vi "Facade.vi"(0 "Data In":T10 {"Input sources" items=["--unused--", "Probe Mic Right", "Probe Mic Left", "Cal Mic", "ABR", "CAP Right", "CAP Left", "Startle piezo", "Temperature", "Heart rate", "Accelerometer", "Startle piezo 2"]; "Output sources" items=["--unused--", "Right primary", "Right secondary", "Left primary", "Left secondary", "Shocks", "Startle", "Background", "Shaker", "Blue laser"]}, 2 "Display State In":T7, 3 "Container State":T9) -> (6 "Data Out":T10 {"Input sources" items=["--unused--", "Probe Mic Right", "Probe Mic Left", "Cal Mic", "ABR", "CAP Right", "CAP Left", "Startle piezo", "Temperature", "Heart rate", "Accelerometer", "Startle piezo 2"]; "Output sources" items=["--unused--", "Right primary", "Right secondary", "Left primary", "Left secondary", "Shocks", "Startle", "Background", "Shaker", "Blue laser"]}, 7 "Display State Out":T7, 8 "Action":T6)   [LabVIEW 2020, in "PXISlot.xctl"]
uses:
  PXISlot.xctl
  Input sources.ctl
  Output sources.ctl
  Data.ctl
  <vilib>/_xctls/Container State.ctl
  State.ctl
  Connector Type.ctl
  <vilib>/_xctls/Action.ctl
  <vilib>/_xctls/XControlSupport.lvlib
panel:
  in  "PXISlot Control":T1(tab) caption="SLOT X"
  in  "PXI-4461":cluster{"AI0":T2, "AO0":T3, "AO1":T3, "AI1":T2} caption="Slot X" {"AI1" items=["--unused--", "Probe Mic Right", "Probe Mic Left", "Cal Mic", "ABR", "CAP Right", "CAP Left", "Startle piezo", "Temperature", "Heart rate", "Accelerometer", "Startle piezo 2"]; "AO1" items=["--unused--", "Right primary", "Right secondary", "Left primary", "Left secondary", "Shocks", "Startle", "Background", "Shaker", "Blue laser"]; "AO0" items=["--unused--", "Right primary", "Right secondary", "Left primary", "Left secondary", "Shocks", "Startle", "Background", "Shaker", "Blue laser"]; "AI0" items=["--unused--", "Probe Mic Right", "Probe Mic Left", "Cal Mic", "ABR", "CAP Right", "CAP Left", "Startle piezo", "Temperature", "Heart rate", "Accelerometer", "Startle piezo 2"]}
  in  "BNC-2110":T4 caption="Slot X" {"AI7" items=["--unused--", "Probe Mic Right", "Probe Mic Left", "Cal Mic", "ABR", "CAP Right", "CAP Left", "Startle piezo", "Temperature", "Heart rate", "Accelerometer", "Startle piezo 2"]; "AI6" items=["--unused--", "Probe Mic Right", "Probe Mic Left", "Cal Mic", "ABR", "CAP Right", "CAP Left", "Startle piezo", "Temperature", "Heart rate", "Accelerometer", "Startle piezo 2"]; "AI5" items=["--unused--", "Probe Mic Right", "Probe Mic Left", "Cal Mic", "ABR", "CAP Right", "CAP Left", "Startle piezo", "Temperature", "Heart rate", "Accelerometer", "Startle piezo 2"]; "AI4" items=["--unused--", "Probe Mic Right", "Probe Mic Left", "Cal Mic", "ABR", "CAP Right", "CAP Left", "Startle piezo", "Temperature", "Heart rate", "Accelerometer", "Startle piezo 2"]; "AI3" items=["--unused--", "Probe Mic Right", "Probe Mic Left", "Cal Mic", "ABR", "CAP Right", "CAP Left", "Startle piezo", "Temperature", "Heart rate", "Accelerometer", "Startle piezo 2"]; "AI2" items=["--unused--", "Probe Mic Right", "Probe Mic Left", "Cal Mic", "ABR", "CAP Right", "CAP Left", "Startle piezo", "Temperature", "Heart rate", "Accelerometer", "Startle piezo 2"]; "AI1" items=["--unused--", "Probe Mic Right", "Probe Mic Left", "Cal Mic", "ABR", "CAP Right", "CAP Left", "Startle piezo", "Temperature", "Heart rate", "Accelerometer", "Startle piezo 2"]; "AO0" items=["--unused--", "Right primary", "Right secondary", "Left primary", "Left secondary", "Shocks", "Startle", "Background", "Shaker", "Blue laser"]; "AO1" items=["--unused--", "Right primary", "Right secondary", "Left primary", "Left secondary", "Shocks", "Startle", "Background", "Shaker", "Blue laser"]; "AI0" items=["--unused--", "Probe Mic Right", "Probe Mic Left", "Cal Mic", "ABR", "CAP Right", "CAP Left", "Startle piezo", "Temperature", "Heart rate", "Accelerometer", "Startle piezo 2"]}
  in  "BNC-2090":T5 caption="Slot X" {"AI7" items=["--unused--", "Probe Mic Right", "Probe Mic Left", "Cal Mic", "ABR", "CAP Right", "CAP Left", "Startle piezo", "Temperature", "Heart rate", "Accelerometer", "Startle piezo 2"]; "AI5" items=["--unused--", "Probe Mic Right", "Probe Mic Left", "Cal Mic", "ABR", "CAP Right", "CAP Left", "Startle piezo", "Temperature", "Heart rate", "Accelerometer", "Startle piezo 2"]; "AI3" items=["--unused--", "Probe Mic Right", "Probe Mic Left", "Cal Mic", "ABR", "CAP Right", "CAP Left", "Startle piezo", "Temperature", "Heart rate", "Accelerometer", "Startle piezo 2"]; "AI1" items=["--unused--", "Probe Mic Right", "Probe Mic Left", "Cal Mic", "ABR", "CAP Right", "CAP Left", "Startle piezo", "Temperature", "Heart rate", "Accelerometer", "Startle piezo 2"]; "AI6" items=["--unused--", "Probe Mic Right", "Probe Mic Left", "Cal Mic", "ABR", "CAP Right", "CAP Left", "Startle piezo", "Temperature", "Heart rate", "Accelerometer", "Startle piezo 2"]; "AI4" items=["--unused--", "Probe Mic Right", "Probe Mic Left", "Cal Mic", "ABR", "CAP Right", "CAP Left", "Startle piezo", "Temperature", "Heart rate", "Accelerometer", "Startle piezo 2"]; "AO1" items=["--unused--", "Right primary", "Right secondary", "Left primary", "Left secondary", "Shocks", "Startle", "Background", "Shaker", "Blue laser"]; "AI2" items=["--unused--", "Probe Mic Right", "Probe Mic Left", "Cal Mic", "ABR", "CAP Right", "CAP Left", "Startle piezo", "Temperature", "Heart rate", "Accelerometer", "Startle piezo 2"]; "AO0" items=["--unused--", "Right primary", "Right secondary", "Left primary", "Left secondary", "Shocks", "Startle", "Background", "Shaker", "Blue laser"]; "AI0" items=["--unused--", "Probe Mic Right", "Probe Mic Left", "Cal Mic", "ABR", "CAP Right", "CAP Left", "Startle piezo", "Temperature", "Heart rate", "Accelerometer", "Startle piezo 2"]}
  in  "PXIe-4463":cluster{"AO0":T3, "AO1":T3} caption="Slot X" {"AO1" items=["--unused--", "Right primary", "Right secondary", "Left primary", "Left secondary", "Shocks", "Startle", "Background", "Shaker", "Blue laser"]; "AO0" items=["--unused--", "Right primary", "Right secondary", "Left primary", "Left secondary", "Shocks", "Startle", "Background", "Shaker", "Blue laser"]}
  in  "PXIe-4464":cluster{"AI0":T2, "AI1":T2, "AI2":T2, "AI3":T2} caption="Slot X" {"AI3" items=["--unused--", "Probe Mic Right", "Probe Mic Left", "Cal Mic", "ABR", "CAP Right", "CAP Left", "Startle piezo", "Temperature", "Heart rate", "Accelerometer", "Startle piezo 2"]; "AI2" items=["--unused--", "Probe Mic Right", "Probe Mic Left", "Cal Mic", "ABR", "CAP Right", "CAP Left", "Startle piezo", "Temperature", "Heart rate", "Accelerometer", "Startle piezo 2"]; "AI1" items=["--unused--", "Probe Mic Right", "Probe Mic Left", "Cal Mic", "ABR", "CAP Right", "CAP Left", "Startle piezo", "Temperature", "Heart rate", "Accelerometer", "Startle piezo 2"]; "AI0" items=["--unused--", "Probe Mic Right", "Probe Mic Left", "Cal Mic", "ABR", "CAP Right", "CAP Left", "Startle piezo", "Temperature", "Heart rate", "Accelerometer", "Startle piezo 2"]}
types:
  T1 = enum32{"None", "PXI-4461", "BNC-2110", "BNC-2090", "PXIe-4463", "PXIe-4464"}
  T2 = typedef "Input sources.ctl" = u16
  T3 = typedef "Output sources.ctl" = u16
  T4 = cluster{"AI0":T2, "AO1":T3, "AO0":T3, "AI1":T2, "AI2":T2, "AI3":T2, "AI4":T2, "AI5":T2, "AI6":T2, "AI7":T2, "Trigger":string}
  T5 = cluster{"AI0":T2, "AO0":T3, "AI2":T2, "AO1":T3, "AI4":T2, "AI6":T2, "AI1":T2, "AI3":T2, "AI5":T2, "AI7":T2, "Trigger":string}
  T6 = typedef "XControlSupport.lvlib/Action.ctl" = cluster{"Data Changed?":bool, "State Changed?":bool, "Action Name":string}
  T7 = typedef "PXISlot.xctl/State.ctl" = cluster{"Connector Type":T8, "Hide unused":bool, "Type change?":bool, "Is dirty?":bool, "SlotNum":i32, "Trigger Visible":bool}
  T8 = typedef "Connector Type.ctl" = enum16{"None", "PXI-4461", "BNC-2110", "BNC-2090", "PXIe-4463", "PXIe-4464"}
  T9 = typedef "XControlSupport.lvlib/Container State.ctl" = cluster{"Indicator?":bool, "Run Mode?":bool, " Refnum":refnum<vi>}
  T10 = typedef "PXISlot.xctl/Data.ctl" = cluster{"Output sources":T3[], "Input sources":T2[]}
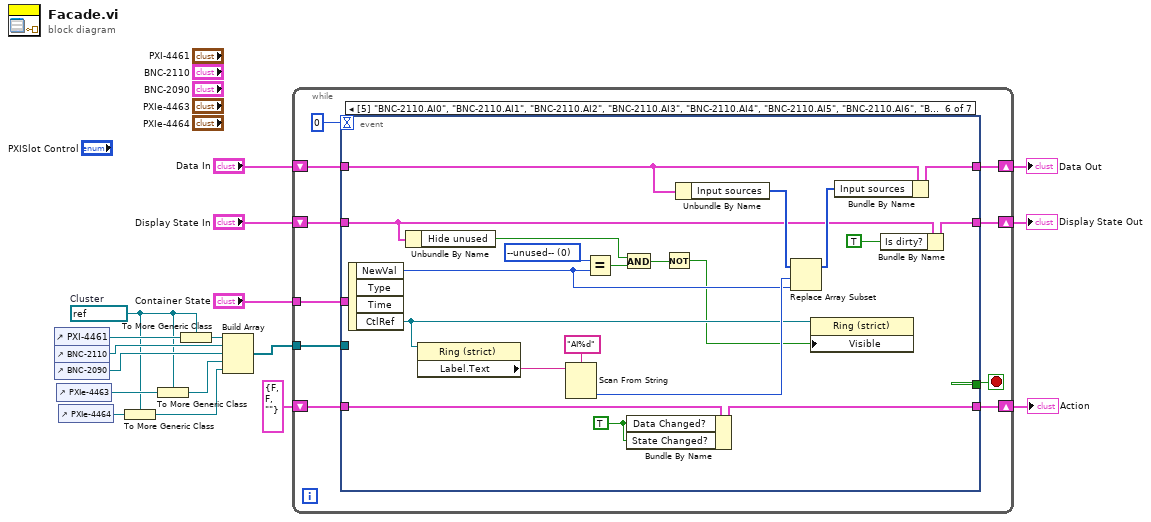
[diagram p0: block diagram]
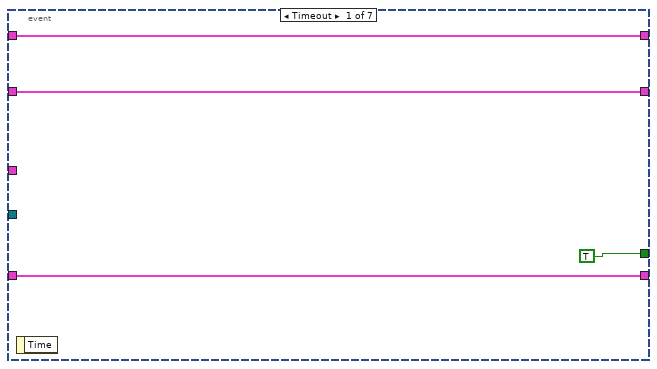
[diagram p2: hidden frame]
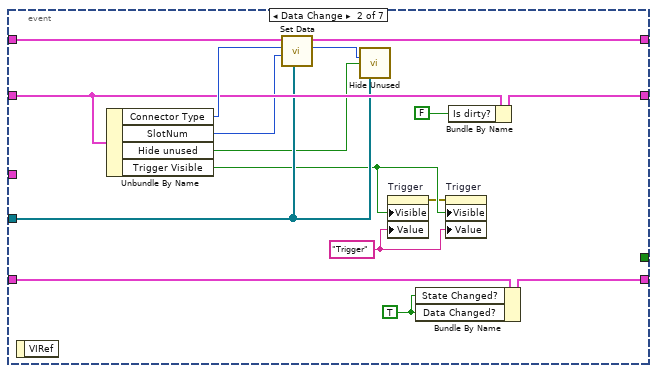
[diagram p3: hidden frame]
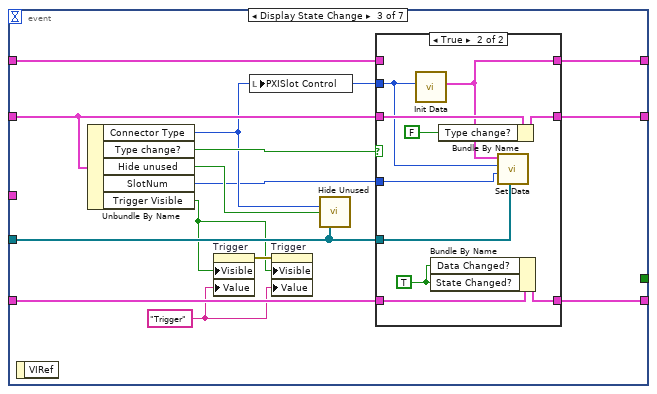
[diagram p4: hidden frame]
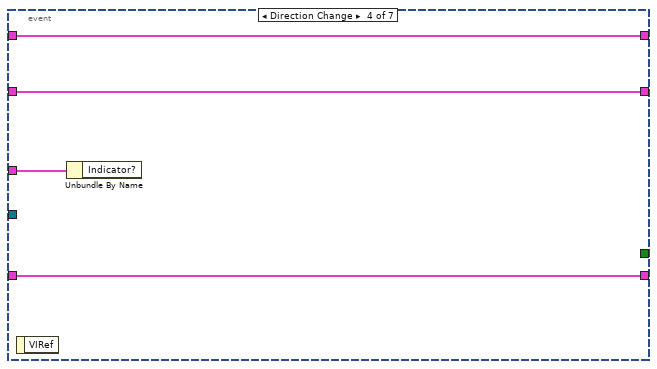
[diagram p6: hidden frame]
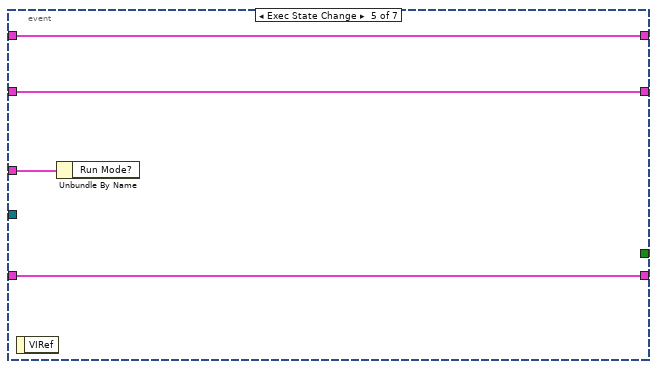
[diagram p7: hidden frame]
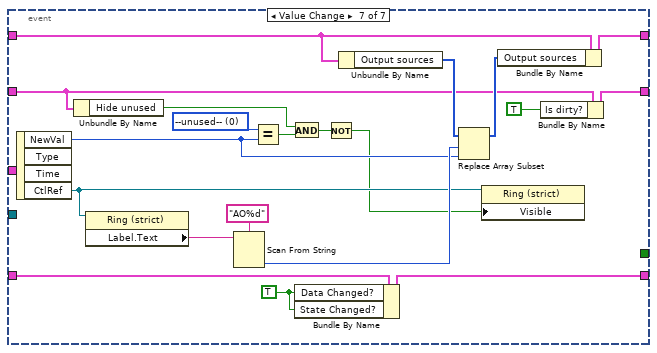
[diagram p8: hidden frame]
diagram:
  w1 = refnum<vi> refnum  # Cluster
  n1 = control-ref of="PXI-4461"() -> (w10:refnum<vi>)
  n2 = control-ref of="BNC-2110"() -> (w9:refnum<vi>)
  n3 = control-ref of="BNC-2090"() -> (w8:refnum<vi>)
  n4 = control-ref of="PXIe-4463"() -> (w5:refnum<vi>)
  n5 = control-ref of="PXIe-4464"() -> (w3:refnum<vi>)
  n6 = To More Generic Class(target class=w1, reference=w3) -> (generic class reference=w2:refnum<vi>)
  n7 = To More Generic Class(target class=w1, reference=w5) -> (generic class reference=w4:refnum<vi>)
  n8 = To More Generic Class(target class=w1, reference=w10) -> (generic class reference=w6:refnum<vi>)
  n9 = Build Array(w6, w9, w8, w4, w2) -> (w7:refnum<vi>[])
  n10 = while {
    shift-right: [w26] -> w14
    shift-left: "Display State In" -> [w27]
    tunnel: "Container State" -> [w23]
    shift-right: [w21] -> w17
    shift-left: "Data In" -> [w22]
    shift-right: [w19] -> w12
    shift-left: T6 {"Data Changed?"=FALSE, "State Changed?"=FALSE, "Action Name"=""} ("Action") -> [w20]
    tunnel: w7 -> [w18]
    stop <- w25 stop-if-true
    n11 = event shown="[5] \"BNC-2110.AI0\", \"BNC-2110.AI1\", \"BNC-2110.AI2\", \"BNC-2110.AI3\", \"BNC-2110.AI4\", \"BNC-2110.AI5\", \"BNC-2110.AI6\", \"BNC-2110.AI7\", \"PXI-4461.AI0\", \"PXI-4461.AI1\", \"BNC-2090.AI0\", \"BNC-2090.AI1\", \"BNC-2090.AI2\", \"BNC-2090.AI3\", \"BNC-2090.AI4\", \"BNC-2090.AI5\", \"BNC-2090.AI6\", \"BNC-2090.AI7\", \"PXIe-4464.AI0\", \"PXIe-4464.AI1\", \"PXIe-4464.AI2\", \"PXIe-4464.AI3\": Value Change" {
      selector: _ -> [_ _ _ _ _ _ _]
      dyn-events: _ -> [_ _ _ _ _ _ _]
      timeout: 0 -> [_ _ _ _ _ _ _]
      tunnel: w27 -> [w29 w40 w59 w77 w81 w84 w104]
      tunnel: [w29 w38 w58 w77 w81 w83 w103] -> w26
      tunnel: [TRUE _ _ _ _ _ _] -> w25
      tunnel: w23 -> [_ _ _ w78 w82 _ _]
      tunnel: w22 -> [w28 w47 w55 w76 w80 w101 w121]
      tunnel: [w28 w46 w54 w76 w80 w99 w119] -> w21
      tunnel: [w30 w43 w56 w75 w79 w97 w117] -> w19
      tunnel: w20 -> [w30 w44 w57 w75 w79 w98 w118]
      tunnel: w18 -> [_ w37 w52 _ _ _ _]
      event Timeout {
        n12 = event-data() -> ()  [unwired: 1 in, 1 out]
      }
      event Data Change {
        w32 = "Trigger" ("Value")
        w41 = TRUE ("Data Changed?")
        n13 = event-data() -> ()  [unwired: 1 in, 1 out]
        n14 = Unbundle By Name(w40) -> ("Connector Type"=w45:T8, "SlotNum"=w36:i32, "Hide unused"=w35:bool, "Trigger Visible"=w34:bool)
        n15 = call "Set Data.vi"("Connector array"=w37, "SlotNum"=w36, "Connector Type"=w45, "Data"=w47) -> ("Connector Type out"=w42:T8, "Data out"=w46:T10)  [unwired: 6 in]
        n16 = call "Hide Unused.vi"("Connector Type"=w42, "Hide unused"=w35, "Connector array"=w37) -> ()  [unwired: 13 in]
        n17 = property on="Trigger" class="Str"("Visible"=w34, "Value"=w32) -> (error out=w33:errorcluster)  [unwired: 2 in, 1 out]
        n18 = Bundle By Name(cluster=w44, "State Changed?"=w41, "Data Changed?"=w41) -> (w43:T6)
        n19 = property on="Trigger" class="Str"(error in=w33, "Visible"=w34, "Value"=w32) -> ()  [unwired: 1 in, 2 out]
        n20 = Bundle By Name(cluster=w40, "Is dirty?"=FALSE) -> (w38:T7)
      }
      event Display State Change {
        w50 = "Trigger" ("Value")
        n21 = event-data() -> ()  [unwired: 1 in, 1 out]
        n22 = Unbundle By Name(w59) -> ("Connector Type"=w53:T8, "Type change?"=w60:bool, "Hide unused"=w61:bool, "SlotNum"=w51:i32, "Trigger Visible"=w48:bool)
        n23 = property on="Trigger" class="Str"("Visible"=w48, "Value"=w50) -> (error out=w49:errorcluster)  [unwired: 2 in, 1 out]
        n24 = local write "PXISlot Control"(w53) -> ()
        n25 = property on="Trigger" class="Str"(error in=w49, "Visible"=w48, "Value"=w50) -> ()  [unwired: 1 in, 2 out]
        n26 = call "Hide Unused.vi"("Connector Type"=w53, "Hide unused"=w61, "Connector array"=w52) -> ()  [unwired: 13 in]
        n27 = case shown="True" w60 {
          tunnel: w59 -> [w64 w74]
          tunnel: [w64 w73] -> w58
          tunnel: w57 -> [w63 w71]
          tunnel: [w63 w70] -> w56
          tunnel: w55 -> [w62 _]
          tunnel: [w62 w68] -> w54
          tunnel: w53 -> [_ w67]
          tunnel: w52 -> [_ w66]
          tunnel: w51 -> [_ w65]
          frame False {
          }
          frame True {
            w69 = TRUE ("State Changed?")
            n28 = call "Init Data.vi"("Connector Type"=w67) -> ("Data"=w68:T10)  [unwired: 10 in]
            n29 = Bundle By Name(cluster=w71, "Data Changed?"=w69, "State Changed?"=w69) -> (w70:T6)
            n30 = Bundle By Name(cluster=w74, "Type change?"=FALSE) -> (w73:T7)
            n31 = call "Set Data.vi"("Connector array"=w66, "SlotNum"=w65, "Connector Type"=w67, "Data"=w68) -> ()  [unwired: 6 in, 2 out]
          }
        }
      }
      event Direction Change {
        n32 = event-data() -> ()  [unwired: 1 in, 1 out]
        n33 = Unbundle By Name(w78) -> ()  [unwired: 1 out]
      }
      event Exec State Change {
        n34 = event-data() -> ()  [unwired: 1 in, 1 out]
        n35 = Unbundle By Name(w82) -> ()  [unwired: 1 out]
      }
      event Value Change {
        w89 = T2 0 items=["--unused--", "Probe Mic Right", "Probe Mic Left", "Cal Mic", "ABR", "CAP Right", "CAP Left", "Startle piezo", "Temperature", "Heart rate"] ("y")
        w86 = TRUE ("Data Changed?")
        n36 = event-data() -> ("NewVal"=w88:T2, "CtlRef"=w91:refnum<vi>)  [unwired: 1 in, 2 out]
        n37 = Unbundle By Name(w84) -> ("Hide unused"=w92:bool)
        n38 = property class="Ring (strict)"(reference=w91) -> ("Label.Text"=w96:string)  [unwired: 1 in, 2 out]
        n39 = Scan From String(format string="AI%d", input string=w96) -> (output 1=w94:i32)  [unwired: 3 in, 3 out]
        n40 = Equal?(x=w89, y=w88) -> (x = y?=w93:bool)
        n41 = And(x=w92, y=w93) -> (x .and. y?=w90:bool)
        n42 = Bundle By Name(cluster=w98, "Data Changed?"=w86, "State Changed?"=w86) -> (w97:T6)
        n43 = Not(x=w90) -> (.not. x?=w87:bool)
        n44 = Unbundle By Name(w101) -> ("Input sources"=w102:T2[])
        n45 = Replace Array Subset(array=w102, new element=w88, index=w94) -> (w100:T2[])
        n46 = property class="Ring (strict)"(reference=w91, "Visible"=w87) -> ()  [unwired: 1 in, 2 out]
        n47 = Bundle By Name(cluster=w101, "Input sources"=w100) -> (w99:T10)
        n48 = Bundle By Name(cluster=w84, "Is dirty?"=TRUE) -> (w83:T7)
      }
      event Value Change {
        w109 = T3 0 items=["--unused--", "Right primary", "Right secondary", "Left primary", "Left secondary", "Shocks", "Startle", "Background"] ("y")
        w105 = TRUE ("Data Changed?")
        n49 = event-data() -> ("NewVal"=w108:T3, "CtlRef"=w111:refnum<vi>)  [unwired: 1 in, 2 out]
        n50 = Unbundle By Name(w104) -> ("Hide unused"=w112:bool)
        n51 = property class="Ring (strict)"(reference=w111) -> ("Label.Text"=w116:string)  [unwired: 1 in, 2 out]
        n52 = Scan From String(format string="AO%d", input string=w116) -> (output 1=w114:i32)  [unwired: 3 in, 3 out]
        n53 = Equal?(x=w109, y=w108) -> (x = y?=w113:bool)
        n54 = And(x=w112, y=w113) -> (x .and. y?=w110:bool)
        n55 = Bundle By Name(cluster=w118, "Data Changed?"=w105, "State Changed?"=w105) -> (w117:T6)
        n56 = Not(x=w110) -> (.not. x?=w107:bool)
        n57 = Unbundle By Name(w121) -> ("Output sources"=w122:T3[])
        n58 = Replace Array Subset(array=w122, new element=w108, index=w114) -> (w120:T3[])
        n59 = property class="Ring (strict)"(reference=w111, "Visible"=w107) -> ()  [unwired: 1 in, 2 out]
        n60 = Bundle By Name(cluster=w121, "Output sources"=w120) -> (w119:T10)
        n61 = Bundle By Name(cluster=w104, "Is dirty?"=TRUE) -> (w103:T7)
      }
    }
  }
  "Display State Out" <- w14
  "Data Out" <- w17
  "Action" <- w12
